vi "hideCaption&Label.vi"(8 "error in (no error)":errorcluster, 11 "Control in":refnum<vi>) -> (0 "error out":errorcluster, 1 "Label.Visible":bool, 2 "Caption.Visible":bool, 3 "Control out":refnum<vi>)   [LabVIEW 2023]
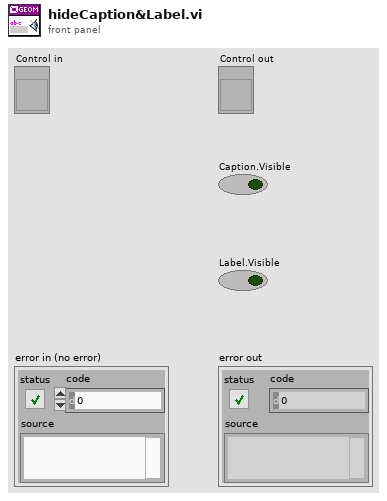
[diagram p1: front panel]
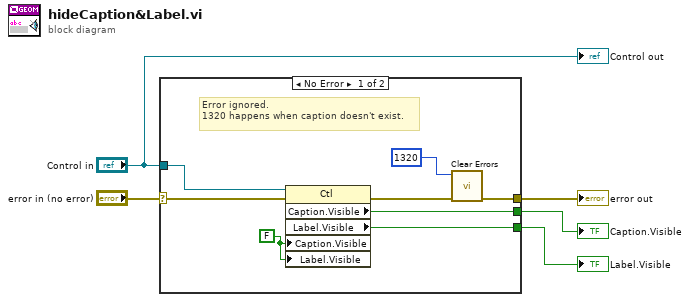
[diagram p0: block diagram]
diagram:
  n1 = case shown="No Error" "error in (no error)" {
    selector: "error in (no error)" -> [w11 w14]
    tunnel: [w7 w14] -> w4
    tunnel: [w10 _] -> w3
    tunnel: [w9 _] -> w2
    tunnel: "Control in" -> [w8 _]
    frame No Error {
      w12 = FALSE ("Caption.Visible")
      # "Error ignored.\n1320 happens when caption doesn't exist."
      n2 = property class="Ctl"(reference=w8, error in=w11, "Caption.Visible"=w12, "Label.Visible"=w12) -> (error out=w13:errorcluster, "Caption.Visible"=w10:bool, "Label.Visible"=w9:bool)  [unwired: 1 out]
      n3 = call <vilib>:"Clear Errors.vi"("error in (no error)"=w13, "specific error code to clear (0: all)"=1320) -> ("error out"=w7:errorcluster)  [unwired: 4 in, 1 out]
    }
    frame Error {
    }
  }
  "Label.Visible" <- w2
  "Caption.Visible" <- w3
  "error out" <- w4
  "Control out" <- "Control in"
